vi "simx Erase File.vi"(8 "error in (no error)":errorcluster, 9 "operationMode":i32, 10 "fileName_serverSide":string, 11 "clientID":i32) -> (0 "error out":errorcluster, 3 "function return":i32)   [LabVIEW 2019, in "PXL_V-REP.lvlib"]
doc: "EXTAPI_DLLEXPORT simxInt simxEraseFile(simxInt clientID,const simxChar* fileName_serverSide,simxInt operationMode);"
uses:
  PXL_V-REP.lvlib
  <userlib>/V-REP/remoteApi.dll
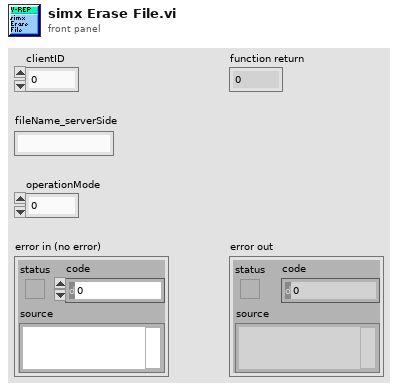
[diagram p1: front panel]
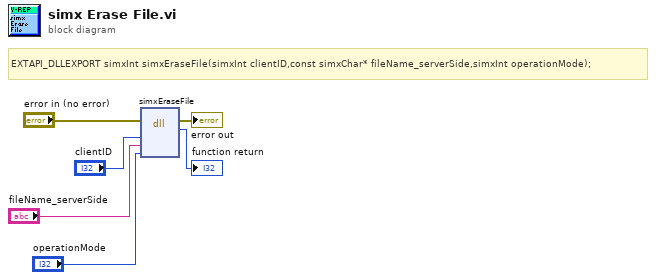
[diagram p0: block diagram]
diagram:
  # "EXTAPI_DLLEXPORT simxInt simxEraseFile(simxInt clientID,const simxChar* fileName_serverSide,simxInt operationMode);"
  n1 = dll-call lib="C:/Program Files (x86)/National Instruments/LabVIEW 2019/user.lib/V-REP/remoteApi.*" fn="simxEraseFile"(error in="error in (no error)", "clientID"="clientID", "fileName_serverSide"="fileName_serverSide", "operationMode"="operationMode") -> (error out=→"error out":errorcluster, →"function return":i32)  [unwired: 5 in, 1 out]
